vi "Read rotPA.vi"(8 "error in (no error)":errorcluster, 11 "RotatorPositions in":refnum<class "RotatorPositions.lvclass">) -> (0 "error out":errorcluster, 2 "rotPA":dbl[unit] min=0.0 max=6.283185307179586, 3 "RotatorPositions out":refnum<class "RotatorPositions.lvclass">)   [LabVIEW 2022 SP3, in "TCSDataDefinitions.lvlib" / "TCSPublicStatus.lvlib" / "PointingPositions.lvlib" / "RotatorPositions.lvclass"]
uses:
  RotatorPositions.lvclass
  RotatorPositions.lvclass/RotatorPositions.ctl
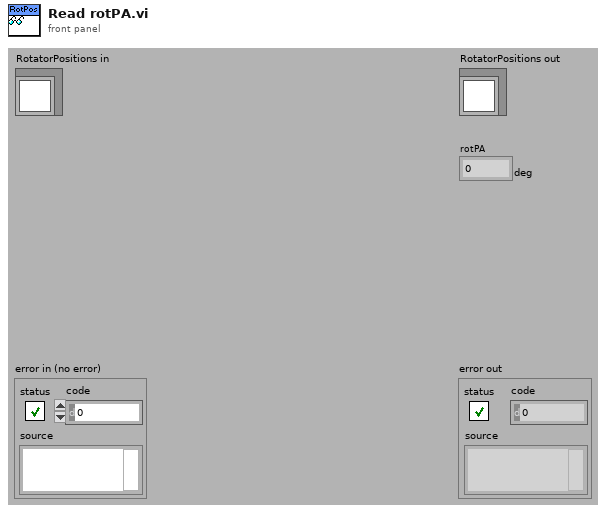
[diagram p1: front panel]
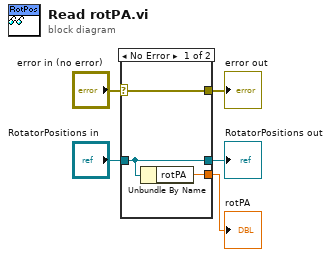
[diagram p0: block diagram]
diagram:
  n1 = case shown="No Error" "error in (no error)" {
    selector: "error in (no error)" -> [w8 w9]
    tunnel: [w8 w9] -> w4
    tunnel: [w7 w10] -> w2
    tunnel: "RotatorPositions in" -> [w7 w10]
    tunnel: [w6 _] -> w1
    frame No Error {
      n2 = Unbundle By Name(w7) -> ("rotPA"=w6:dbl[unit])
    }
    frame Error {
    }
  }
  "error out" <- w4
  "RotatorPositions out" <- w2
  "rotPA" <- w1
